vi "Create Image Dump.vi"(8 "Error IN":errorcluster, 10 "Controls IN":T2={"TDI Actions"=enum."Set Height", "Width (X)"=[], "Cmd Received?"=FALSE, "Display Height (Y)"=1, "Acquisition Line Rate"=8000.0, "Pixel format"=257, "Binning Horizontal (X)"=1, "Binning Vertical (Y)"=1, "Scan Direction"=0, "TDI Stages"=256, "Reverse X"=FALSE, "Test Pattern"=0, "Running?"=FALSE, "Image Reference"=refnum, "Number of frames"=1, "Segments per Buffer"=1, "Recorded Height"=1, "Display Binning Factor"=1, "File Path"=path "", "Operation mode"=0, "Exposure time (area mode)"=1.0} {"Exposure time (area mode)" min=1.0 max=10000.0; "Operation mode" items=["TDI mode", "Area scan mode"]; "Display Binning Factor" min=1; "Test Pattern" items=["Off", "Grey Horizontal Ramp", "Grey Diagonal Ramp", "Grey Diagonal Ramp Moving"]; "TDI Stages" items=["4"=4, "8"=8, "16"=16, "32"=32, "64"=64, "96"=96, "128"=128, "160"=160, "192"=192, "224"=224, "240"=240, "248"=248, "252"=252, "256"=256]; "Scan Direction" items=["Forward", "Reverse", "LineIn"]; "Binning Vertical (Y)" items=["X1"=1, "X2"=2, "X4"=4, "X8"=8]; "Binning Horizontal (X)" items=["X1"=1, "X2"=2, "X4"=4, "X8"=8]; "Pixel format" items=["Mono8"=257, "Mono10"=258, "Mono12"=259]}) -> (0 "Error OUT":errorcluster, 3 "Image ref OUT":T1)   [LabVIEW 2020]
uses:
  VPD Controls/VPD Note Type.ctl
  VPD Controls/VPD Actions.ctl
  VPD Controls/VPD Pixel format.ctl
  VPD Controls/VPD Binning XX.ctl
  VPD Controls/VPD Scan Direction.ctl
  VPD Controls/VPD TDI Stages.ctl
  VPD Controls/VPD Test Pattern.ctl
  <vilib>/vision/Image Controls.llb/IMAQ Image.ctl
  VPD Controls/VPD Operation mode.ctl
  VPD Controls/VPD Exposure time.ctl
  Cameras/Camera Controls/Camera IMAQ Key Info.ctl
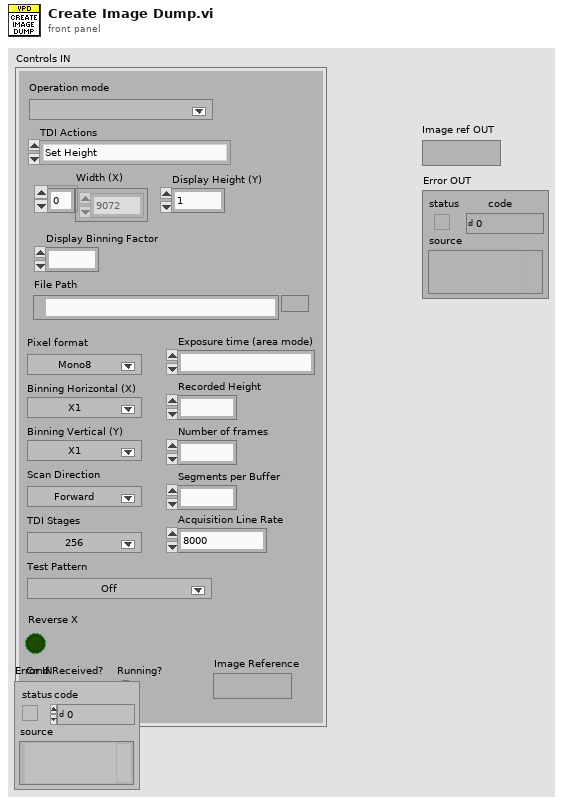
[diagram p1: front panel]
types:
  T1 = typedef "IMAQ Image.ctl" = refnum<image>
  T2 = typedef "VPD Note Type.ctl" = cluster{"TDI Actions":T3, "Width (X)":i64[], "Cmd Received?":bool, "Display Height (Y)":i64, "Acquisition Line Rate":dbl, "Pixel format":T4, "Binning Horizontal (X)":T5, "Binning Vertical (Y)":T5, "Scan Direction":T6, "TDI Stages":T7, "Reverse X":bool, "Test Pattern":T8, "Running?":bool, "Image Reference":T1, "Number of frames":i32, "Segments per Buffer":i64, "Recorded Height":u32, "Display Binning Factor":i32, "File Path":path, "Operation mode":T9, "Exposure time (area mode)":T10}
  T3 = typedef "VPD Actions.ctl" = enum16{"Nothing", "Set Height", "Set ROI", "Set Pixel format", "Set Exposure time", "Set Line rate", "Set Binning Horizontal", "Set Binning Vertical", "Set Scan Direction", "Set TDI Stages", "Set Reverse X", "Set Test Pattern", "Set Segments per Buffer", "Set Operation mode", "Set Display Binning Factor", "Live", "Record", "Quit"}
  T4 = typedef "VPD Pixel format.ctl" = i64
  T5 = typedef "VPD Binning XX.ctl" = u16
  T6 = typedef "VPD Scan Direction.ctl" = i64
  T7 = typedef "VPD TDI Stages.ctl" = u16
  T8 = typedef "VPD Test Pattern.ctl" = u16
  T9 = typedef "VPD Operation mode.ctl" = u16
  T10 = typedef "VPD Exposure time.ctl" = dbl
  T11 = typedef "Camera IMAQ Key Info.ctl" = cluster{"Frame":u32, "Sensor Height":i32, "Sensor Width":i32, "ROI Height":i32, "ROI Width":i32, "ROI Enable?":bool, "Bit per Pixel":u8, "Binning factor":i32}
  T12 = typedef "Image Type" = u32
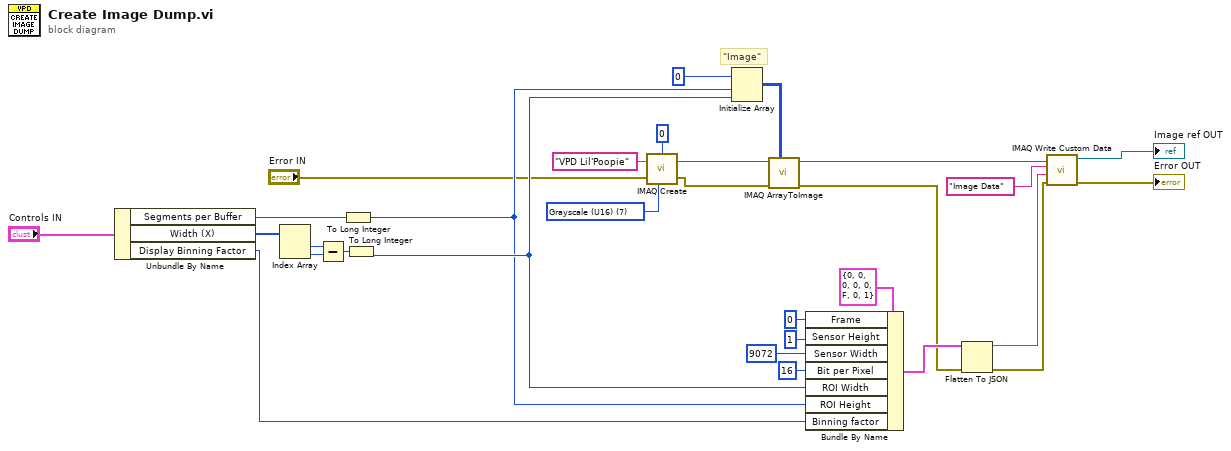
[diagram p0: block diagram]
diagram:
  w25 = T12 7 items=["Grayscale (U8)", "Grayscale (I16)", "Grayscale (SGL)", "Complex (CSG)", "RGB (U32)", "HSL (U32)", "RGB (U64)", "Grayscale (U16)"] ("Image Type")
  # "\"Image\""
  n1 = Unbundle By Name("Controls IN") -> ("Segments per Buffer"=w20:i64, "Width (X)"=w23:i64[], "Display Binning Factor"=w1:i32)
  n2 = Index Array(array=w23) -> (element #1=w21:i64, element #2=w22:i64)  [unwired: 2 in]
  n3 = Subtract(x=w21, y=w22) -> (x-y=w8:i64)
  n4 = To Long Integer(number=w20) -> (32bit integer=w6:i32)
  n5 = To Long Integer(number=w8) -> (32bit integer=w7:i32)
  n6 = call "IMAQ Create"("Border Size"=0, "Image Name"="VPD Lil'Poopie", "Image Type"=w25, "error in (no error)"="Error IN") -> ("New Image"=w26:T1, "error out"=w5:errorcluster)  [unwired: 1 in]
  n7 = Initialize Array(u16 0, w6, w7) -> (w29:u16[][])
  n8 = call "IMAQ ArrayToImage"("Image Pixels (U16)"=w29, "error in (no error)"=w5, "Image"=w26) -> ("error out"=w11:errorcluster, "Image Out"=w12:T1)  [unwired: 7 in]
  n9 = Bundle By Name(cluster=T11 {"Frame"=0, "Sensor Height"=0, "Sensor Width"=0, "ROI Height"=0, "ROI Width"=0, "ROI Enable?"=FALSE, "Bit per Pixel"=0, "Binning factor"=1} ("Camera IMAQ Key Info"), "Frame"=u32 0, "Sensor Height"=1, "Sensor Width"=9072 ("Sensor Height"), "Bit per Pixel"=u8 16, "ROI Width"=w7, "ROI Height"=w6, "Binning factor"=w1) -> (w19:T11)
  n10 = Flatten To JSON(anything=w19, error in (no error)=w11) -> (JSON string=w10:string, 11:w9:errorcluster)  [unwired: 1 in]
  n11 = call "IMAQ Write Custom Data"("error in (no error)"=w9, "Custom Data In"=w10, "Key"="Image Data", "Image"=w12) -> ("error out"=→"Error OUT":errorcluster, "Image Out"=→"Image ref OUT":T1)  [unwired: 6 in]
